vi "SetJSON.vi"(8 "Error In":errorcluster, 9 "Controls?":bool=TRUE, 10 "JSON Input":string, 11 "VI Refnum In":refnum<vi>) -> (0 "Error Out":errorcluster, 3 "VI Refnum Out":refnum<vi>)   [LabVIEW 2019, in "LabJSON.lvlib"]
uses:
  LabJSON.lvlib
  aa3fc0e6-e883-47c7-bda4-2d6daf452595.vi
  <vilib>/JDP Science/JSONtext/JSON text to Variant.vi
  <vilib>/JDP Science/JSONtext/LVClass Serializer/JSONtext LVClass Serializer.lvclass
  <vilib>/JDP Science/JSONtext/JSONtext.lvlib
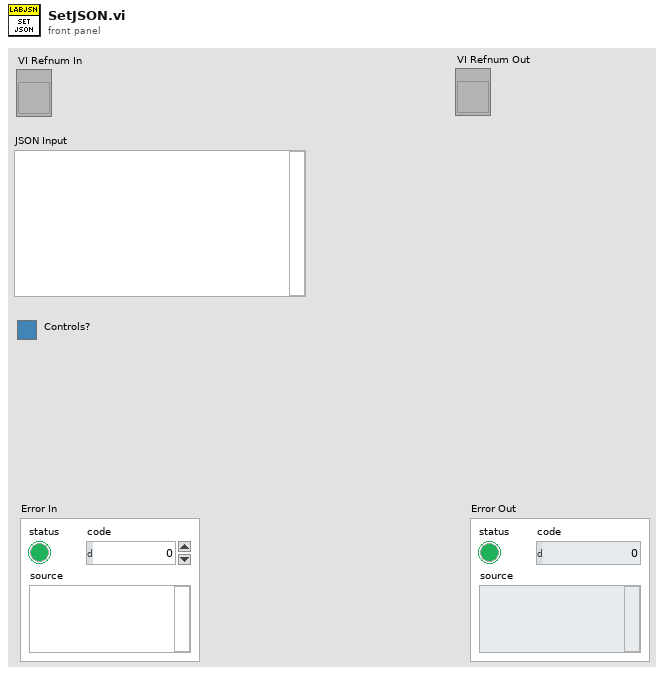
[diagram p1: front panel]
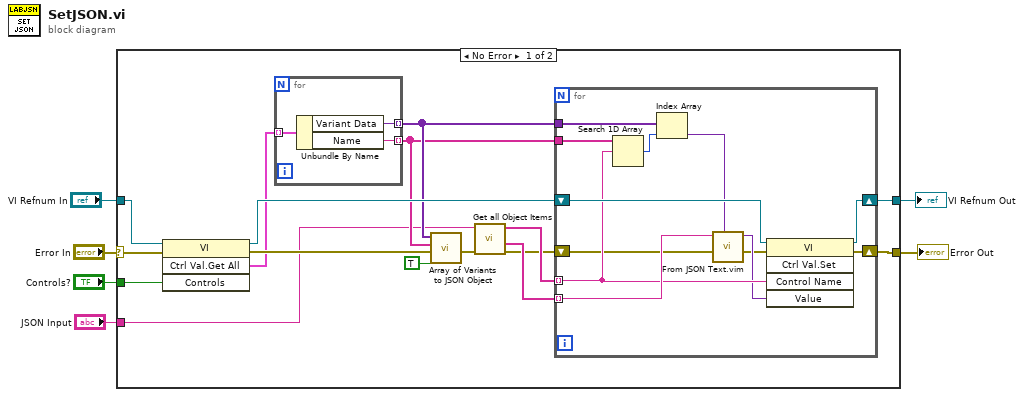
[diagram p0: block diagram]
diagram:
  n1 = case shown="No Error" "Error In" {
    selector: "Error In" -> [w11 w39]
    tunnel: [w9 w39] -> w5
    tunnel: "JSON Input" -> [w10 _]
    tunnel: "VI Refnum In" -> [w12 w38]
    tunnel: [w8 w38] -> w2
    tunnel: "Controls?" -> [w7 _]
    frame No Error {
      n2 = invoke class="VI" method="Ctrl Val.Get All"(reference=w12, error in=w11, "Controls"=w7) -> (reference out=w22:refnum<vi>, error out=w21:errorcluster, "Get All Control Values Variant"=w14:cluster{"Name":string, "Variant Data":variant}[])  [unwired: 1 in, 1 out]
      n3 = for {
        tunnel: w14 -> [w25] mode=indexing
        tunnel: [w24] -> w16 mode=indexing
        tunnel: [w23] -> w15 mode=indexing
        n4 = Unbundle By Name(w25) -> ("Variant Data"=w24:variant, "Name"=w23:string)
      }
      n5 = call <vilib>:"Array of Variants to JSON Object.vi"("Pretty Print?"=TRUE, "error in (no error)"=w21, "Names"=w15, "Array"=w16) -> ("error out"=w17:errorcluster)  [unwired: 6 in, 1 out]
      n6 = call <vilib>:"Get all Object Items.vi"("error in (no error)"=w17, "JSON"=w10) -> ("error out"=w18:errorcluster, "<JSON>"=w19:string[], "Item Names"=w20:string[])  [unwired: 6 in, 1 out]
      n7 = for {
        shift-right: [w35] -> w8
        shift-left: w22 -> [w37]
        shift-right: [w36] -> w9
        shift-left: w18 -> [w27]
        tunnel: w20 -> [w29] mode=indexing
        tunnel: w19 -> [w30] mode=indexing
        tunnel: w15 -> [w34]
        tunnel: w16 -> [w33]
        n8 = Search 1D Array(1D array=w34, element=w29) -> (index of element=w32:i32)  [unwired: 1 in]
        n9 = Index Array(array=w33, index=w32) -> (element=w31:variant)
        n10 = call "From JSON Text.vim"("Data Type and Default Value"=w31, "error in (no error)"=w27, "JSON"=w30) -> ("error out"=w26:errorcluster, "Data out"=w28:variant)  [unwired: 7 in]
        n11 = invoke class="VI" method="Ctrl Val.Set"(reference=w37, error in=w26, "Control Name"=w29, "Value"=w28) -> (reference out=w35:refnum<vi>, error out=w36:errorcluster)  [unwired: 1 in, 3 out]
      }
    }
    frame Error {
    }
  }
  "Error Out" <- w5
  "VI Refnum Out" <- w2
